vi "Fetch Measurement (Others).vi"(8 "error in (no error)":errorcluster, 9 "Timeout (20000 ms)":i32=20000, 10 "Measurement Method (0: Adjacent Channel Power)":u16(ring) items=["Adjacent Channel Power"=0, "Burst Power"=1, "Intermod"=4, "Multi-Carrier Power"=5, "Power State CCDF"=7, "Spurious Emissions"=9], 11 "VISA resource name":refnum<visa-resource-name>) -> (0 "error out":errorcluster, 2 "Measured Values":dbl[](array[numeric]) format="%#.6g", 3 "VISA resource name out":refnum<visa-resource-name>)   [LabVIEW 2014, in "Agilent ESA PSA Series.lvlib"]
doc: "Returns the results of the last measurement( Adjacent Channel Power, Burst Power, Intermod, Multi-Carrier Power, Power State CCDF and Spurious Emissions) and does not initiate data acquisition."
uses:
  Agilent ESA PSA Series.lvlib
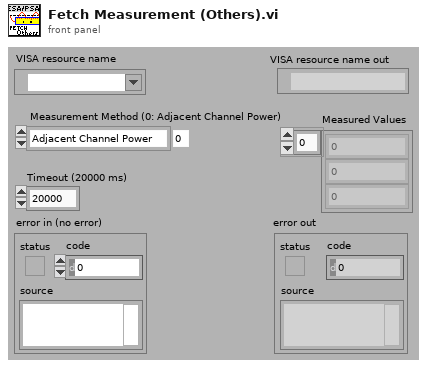
[diagram p1: front panel]
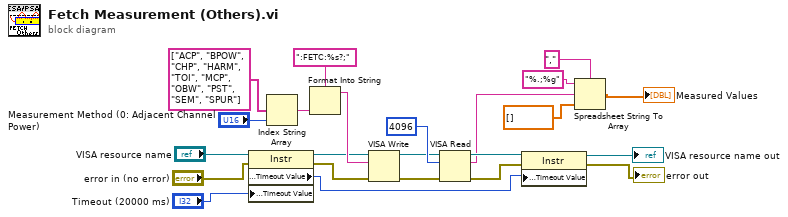
[diagram p0: block diagram]
diagram:
  n1 = property on="Property Node" class="Instr"(reference="VISA resource name", error in="error in (no error)", "General Settings:Timeout Value"="Timeout (20000 ms)") -> (reference out=w12:refnum<visa-resource-name>, error out=w13:errorcluster, "General Settings:Timeout Value"=w9:u32)
  n2 = Index String Array(1:"Measurement Method (0: Adjacent Channel Power)", 2:string[] ["ACP", "BPOW", "CHP", "HARM", "TOI", "MCP", "OBW", "PST", "SEM", "SPUR"]) -> (0:w17:string)  [unwired: 1 in]
  n3 = Format Into String(format string=":FETC:%s?;" ("string (\"\")"), w17) -> (resulting string=w16:string)  [unwired: 2 in, 1 out]
  n4 = VISA Write(VISA resource name=w12, write buffer=w16, error in (no error)=w13) -> (VISA resource name out=w20:refnum<visa-resource-name>, error out=w19:errorcluster)  [unwired: 1 out]
  n5 = VISA Read(VISA resource name=w20, byte count=u32 4096, error in (no error)=w19) -> (VISA resource name out=w11:refnum<visa-resource-name>, read buffer=w1:string, error out=w10:errorcluster)  [unwired: 1 out]
  n6 = property on="Property Node" class="Instr"(reference=w11, error in=w10, "General Settings:Timeout Value"=w9) -> (reference out=→"VISA resource name out":refnum<visa-resource-name>, error out=→"error out":errorcluster)
  n7 = Spreadsheet String To Array(delimiter (Tab)=",", format string="%.;%g", spreadsheet string=w1, array type (2D Dbl)=dbl[] []) -> (array=→"Measured Values":dbl[])
